vi "setup_counter.vi"(8 "error in":errorcluster, 11 "Counter Settings":T2 {"Array of Counter Settings"."Binwidth (ms)" format="%0.2f"}) -> (0 "error out":errorcluster, 3 "Counter Settings, Tasks and Data":T1)   [LabVIEW 2013]
uses:
  <vilib>/DAQmx/create/channels.llb/DAQmx Create Channel (CI-Count Edges).vi
  <vilib>/DAQmx/configure/timing.llb/DAQmx Timing (Sample Clock).vi
  <resource>/objmgr/daqmx.rc
panel:
  in  "Counter Settings, Tasks and Data (in)":T1
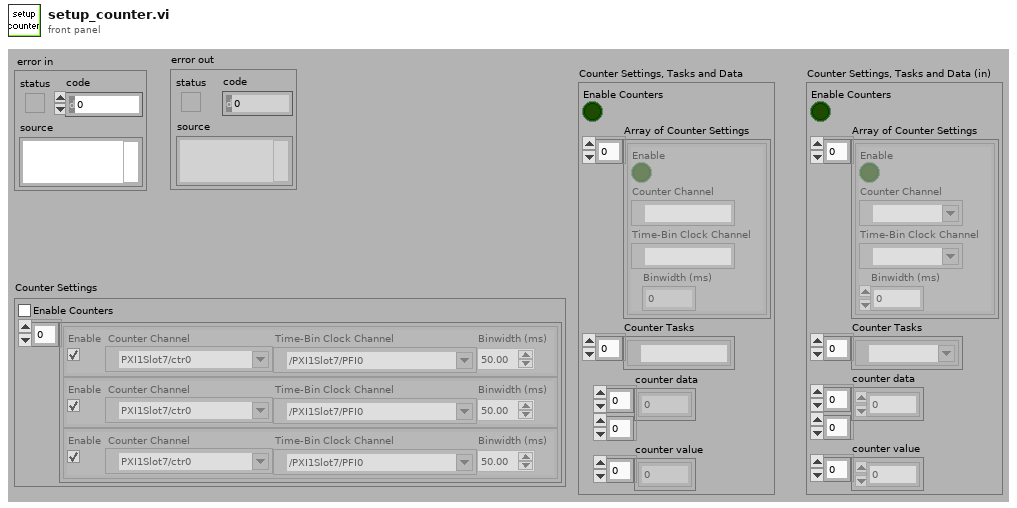
[diagram p1: front panel]
types:
  T1 = cluster{"Enable Counters":bool, "Array of Counter Settings":cluster{"Enable":bool, "Counter Channel":tag, "Time-Bin Clock Channel":tag, "Binwidth (ms)":dbl}[], "Counter Tasks":refnum<k21>[], "counter data":u32[][], "counter value":u32[]}
  T2 = cluster{"Enable Counters":bool, "Array of Counter Settings":cluster{"Enable":bool, "Counter Channel":tag, "Time-Bin Clock Channel":tag, "Binwidth (ms)":dbl}[]}
  T3 = cluster{"Enable":bool, "Counter Channel":tag, "Time-Bin Clock Channel":tag, "Binwidth (ms)":dbl}[]
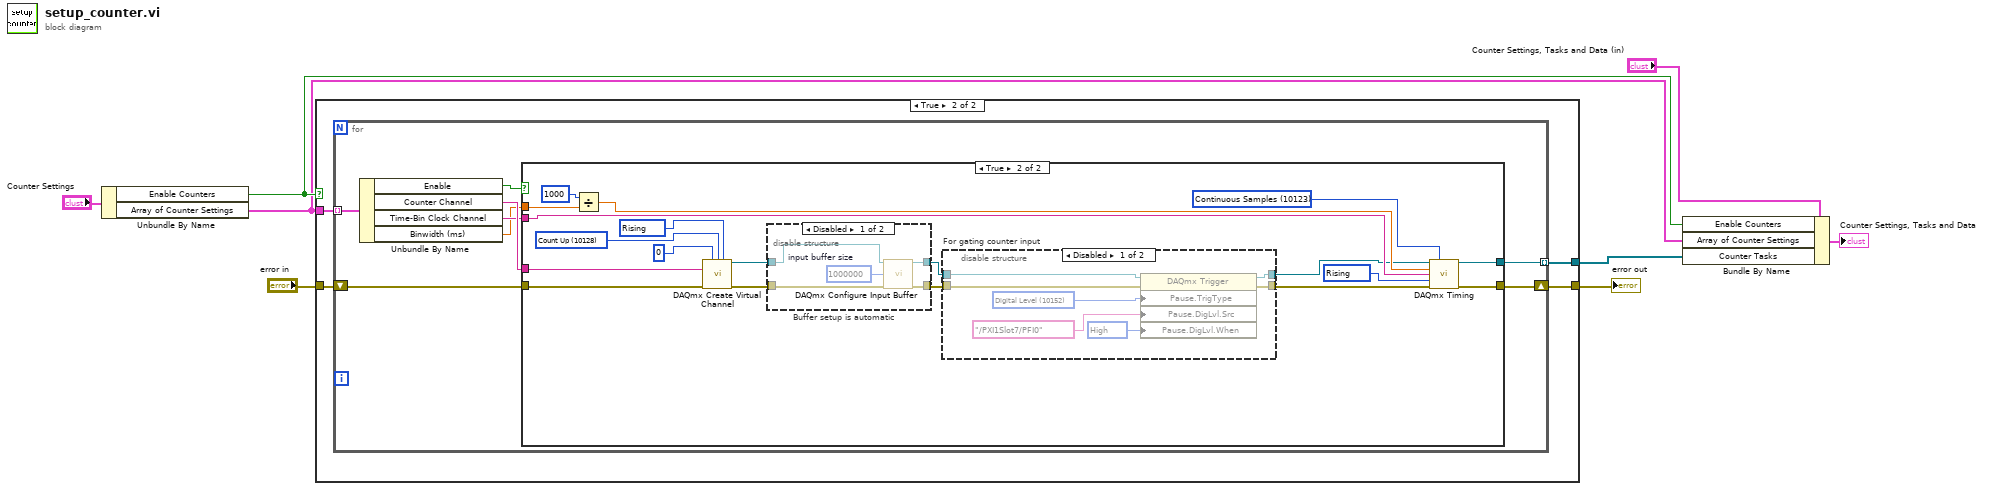
[diagram p0: block diagram]
diagram:
  n1 = Unbundle By Name("Counter Settings") -> ("Enable Counters"=w2:bool, "Array of Counter Settings"=w1:T3)
  n2 = case shown="True" w2 {
    tunnel: "error in" -> [w9 w13]
    tunnel: [w9 w12] -> w7
    tunnel: [_ w11] -> w5
    tunnel: w1 -> [_ w10]
    frame False {
    }
    frame True {
      n3 = for {
        tunnel: w10 -> [w21] mode=indexing
        shift-right: [w15] -> w12
        shift-left: w13 -> [w19]
        tunnel: [w14] -> w11 mode=indexing
        n4 = Unbundle By Name(w21) -> ("Enable"=w20:bool, "Counter Channel"=w18:tag, "Time-Bin Clock Channel"=w17:tag, "Binwidth (ms)"=w16:dbl)
        n5 = case shown="True" w20 {
          tunnel: w19 -> [w22 w32]
          tunnel: w16 -> [_ w31]
          tunnel: [w22 w24] -> w15
          tunnel: w17 -> [_ w30]
          tunnel: w18 -> [_ w29]
          tunnel: [_ w23] -> w14
          frame False {
          }
          frame True {
            w37 = 10280 items=["Rising"=10280, "Falling"=10171] ("active edge")
            w38 = 10123 items=["Finite Samples"=10178, "Continuous Samples"=10123, "Hardware Timed Single Point"=12522] ("sample mode")
            w39 = 10280 items=["Rising"=10280, "Falling"=10171] ("edge")
            w40 = 10128 items=["Count Up"=10128, "Count Down"=10124, "Externally Controlled"=10326] ("count direction")
            n6 = Divide(x=1000, y=w31) -> (x/y=w34:dbl)
            n7 = call-poly <vilib>:"DAQmx Create Virtual Channel.vi"("initial count"=u32 0, "count direction"=w40, "edge"=w39, "counter"=w29, "error in"=w32) -> ("task out"=w36:refnum<k21>, "error out"=w35:errorcluster)  [unwired: 5 in, 4 out]
            n8 = disable-structure "Buffer setup is automatic" shown="Disabled" {
              disable-tunnel: w36 -> [w55 w56]
              disable-tunnel: w35 -> [w54 w57]
              disable-tunnel: [w53 w57] -> w27
              disable-tunnel: [w52 w56] -> w28
              frame Disabled {
                w51 = u32 1000000  # input buffer size
                n9 = call <vilib>:"DAQmx Configure Input Buffer.vi"("task/channels in"=w55, "buffer size (in samples per channel)"=w51, "error in"=w54) -> ("task out"=w52:refnum<k21>, "error out"=w53:errorcluster)  [unwired: 11 out]
              }
              frame Enabled {
              }
            }
            n10 = disable-structure "For gating counter input" shown="Disabled" {
              disable-tunnel: w28 -> [w48 w49]
              disable-tunnel: w27 -> [w47 w50]
              disable-tunnel: [w43 w49] -> w26
              disable-tunnel: [w42 w50] -> w25
              frame Disabled {
                w44 = 10152 items=["Analog Level"=10101, "Analog Window"=10103, "Digital Level"=10152, "Digital Pattern"=10398, "None"=10230] ("Pause.TrigType")
                w46 = 10192 items=["High"=10192, "Low"=10214] ("Pause.DigLvl.When")
                n11 = property class="DAQmx Trigger"(reference=w48, error in=w47, "Pause.TrigType"=w44, "Pause.DigLvl.Src"=tag "/PXI1Slot7/PFI0", "Pause.DigLvl.When"=w46) -> (reference out=w43:refnum<k21>, error out=w42:errorcluster)
              }
              frame Enabled {
              }
            }
            n12 = call-poly <vilib>:"DAQmx Timing.vi"("task/channels in"=w26, "sample mode"=w38, "rate"=w34, "source"=w30, "active edge"=w37, "error in"=w25) -> ("task out"=w23:refnum<k21>, "error out"=w24:errorcluster)  [unwired: 1 in, 7 out]
          }
        }
      }
    }
  }
  "error out" <- w7
  n13 = Bundle By Name(cluster="Counter Settings, Tasks and Data (in)", "Enable Counters"=w2, "Array of Counter Settings"=w1, "Counter Tasks"=w5) -> (→"Counter Settings, Tasks and Data":T1)
